vi "matlabwfexistsdialogue.vi"(1 "Matlab waveform path":path) -> (0 "mtalab waveform path out":path)   [LabVIEW 2015]
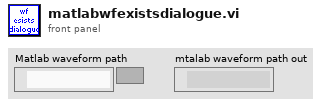
[diagram p1: front panel]
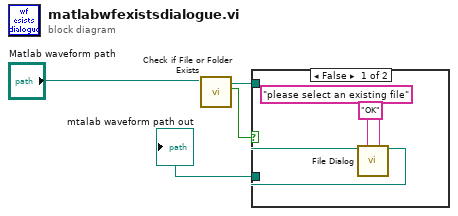
[diagram p0: block diagram]
diagram:
  n1 = call <vilib>:"Check if File or Folder Exists.vi"("path"="Matlab waveform path") -> ("file or folder exists?"=w2:bool, "dup path"=w3:path)  [unwired: 8 in, 1 out]
  n2 = case shown="False" w2 {
    tunnel: [w5 w9] -> w4
    tunnel: w3 -> [w6 w9]
    frame False {
      n3 = call "File Dialog"("start path"=w6, "prompt"="please select an existing file", "button label"="OK") -> ("selected path"=w5:path)  [unwired: 9 in, 3 out]
    }
    frame True {
    }
  }
  "mtalab waveform path out" <- w4
